vi "array -- remove zeros.vi"(8 "array in":dbl[](array[numeric])) -> (0 "Array out":dbl[](array[numeric]))   [LabVIEW 2021]
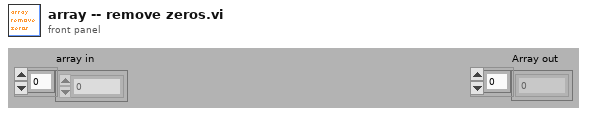
[diagram p1: front panel]
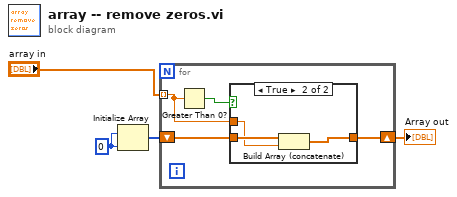
[diagram p0: block diagram]
diagram:
  w4 = 0 ("dimension size")
  n1 = Initialize Array(w4, w4) -> (w3:i32[])
  n2 = for {
    tunnel: "array in" -> [w6] mode=indexing
    shift-right: [w5] -> w1
    shift-left: w3 -> [w7]
    n3 = Greater Than 0?(x=w6) -> (x > 0?=w8:bool)
    n4 = case shown="True" w8 {
      tunnel: w7 -> [w9 w12]
      tunnel: w6 -> [_ w10]
      tunnel: [w9 w11] -> w5
      frame False {
      }
      frame True {
        n5 = Build Array (concatenate)(w12, w10) -> (w11:dbl[])
      }
    }
  }
  "Array out" <- w1
